vi "Execute (Multiple result with rows).vi"(8 "error in (no error)":errorcluster, 10 "SQL":string, 11 "PQ Connection in":refnum<class "PQ Connection.lvclass">) -> (0 "error out":errorcluster, 1 "Results with Rows returned":refnum<class "PQ Result.lvclass">[](array[class]), 3 "PQ Connection out":refnum<class "PQ Connection.lvclass">)   [LabVIEW 2015, in "PQ Connection.lvclass"]
uses:
  PQ Connection.lvclass
  Result/PQ Result.lvclass
  PQ Connection.lvclass/PQ Connection.ctl
  Result/PQ Result.lvclass/PQ Result.ctl
  libpq.dll
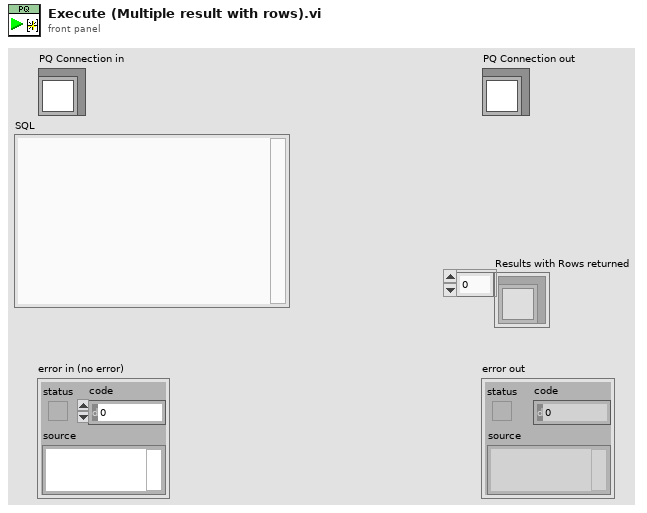
[diagram p1: front panel]
types:
  T1 = typedef "PQ Result.lvclass/Result Status.ctl" = enum32{"PGRES_EMPTY_QUERY", "PGRES_COMMAND_OK", "PGRES_TUPLES_OK", "PGRES_COPY_OUT", "PGRES_COPY_IN", "PGRES_BAD_RESPONSE", "PGRES_NONFATAL_ERROR", "PGRES_FATAL_ERROR", "PGRES_COPY_BOTH", "PGRES_SINGLE_TUPLE"}
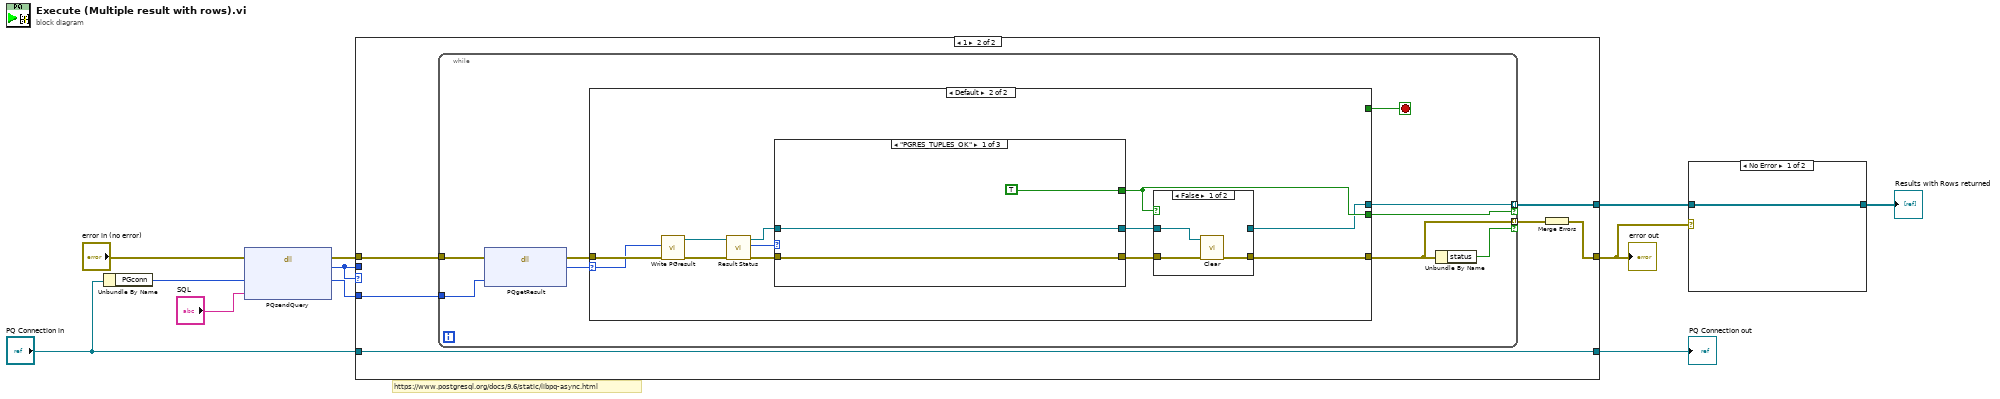
[diagram p0: block diagram]
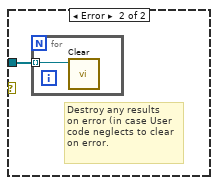
[diagram p2: hidden frame]
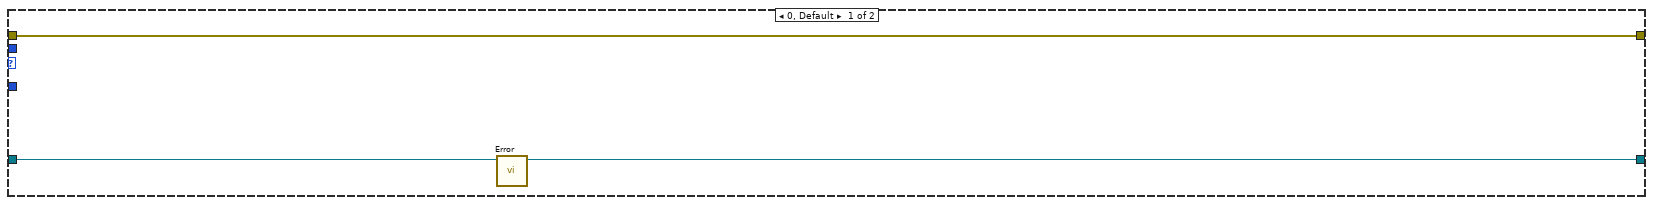
[diagram p3: hidden frame]
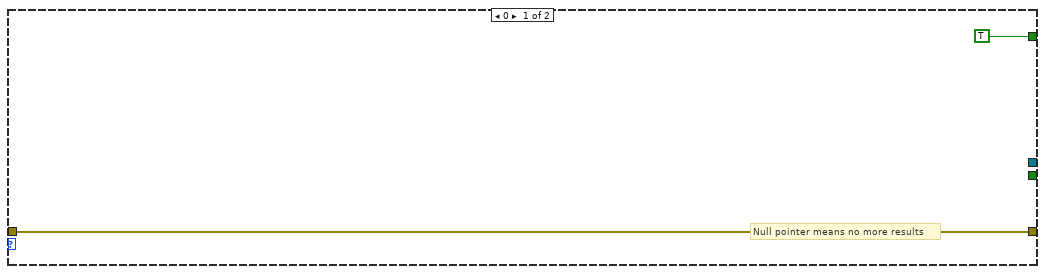
[diagram p4: hidden frame]
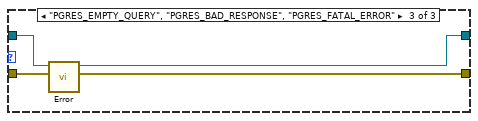
[diagram p6: hidden frame]
diagram:
  # "https://www.postgresql.org/docs/9.6/static/libpq-async.html"
  n1 = Unbundle By Name("PQ Connection in") -> ("PGconn"=w10:u32)
  n2 = dll-call lib="C:/PQ/Connection/libpq.dll" fn="PQsendQuery" ("libpq.*:PQexec")(error in="error in (no error)", "PGconn"=w10, "command"="SQL") -> (error out=w9:errorcluster, "OK?"=w7:u32, "PGconn"=w4:u32)  [unwired: 3 in, 1 out]
  n3 = case shown="1" w7 {
    tunnel: w9 -> [w12 w20]
    tunnel: w7 -> [_ _]
    tunnel: [_ w19] -> w2
    tunnel: [w12 w15] -> w1
    tunnel: "PQ Connection in" -> [w14 w16]
    tunnel: [w13 w16] -> w5
    tunnel: w4 -> [_ w17]
    frame 0, Default {
      n4 = call "Error.vi"("PQ Connection in"=w14) -> ("PQ Connection out"=w13:refnum<class "PQ Connection.lvclass">)  [unwired: 9 in, 1 out]
    }
    frame 1 {
      n5 = while {
        tunnel: [w27] -> w19 mode=indexing if=w28
        tunnel: w17 -> [w29]
        tunnel: w20 -> [w24]
        tunnel: [w22] -> w18 mode=indexing if=w21
        stop <- w25 stop-if-true
        n6 = dll-call lib="C:/PQ/Connection/libpq.dll" fn="PQgetResult" ("libpq.*:PQexec")(error in=w24, "PGconn"=w29) -> (error out=w23:errorcluster, "PQresult"=w26:u32)  [unwired: 3 in, 1 out]
        n7 = case shown="Default" w26 {
          selector: w26 -> [_ w32]
          tunnel: w23 -> [w31 w43]
          tunnel: [_ w42] -> w28
          tunnel: [_ w40] -> w27
          tunnel: [w31 w38] -> w22
          tunnel: [TRUE _] -> w25
          frame 0 {
            # "Null pointer means no more results"
          }
          frame Default {
            n8 = call "Write PGresult.vi"("error in (no error)"=w43, "PGresult"=w32) -> ("error out"=w36:errorcluster, "PQ Result  out"=w37:refnum<class "PQ Result.lvclass">)  [unwired: 8 in]
            n9 = call "Result Status.vi"("error in (no error)"=w36, "PQ Result in"=w37) -> ("error out"=w33:errorcluster, "Result Status"=w35:T1, "PQ Result out"=w34:refnum<class "PQ Result.lvclass">)  [unwired: 7 in]
            n10 = case shown="\"PGRES_TUPLES_OK\"" w35 {
              tunnel: [w45 w47 w49] -> w41
              tunnel: w34 -> [w45 w47 w52]
              tunnel: w33 -> [w46 w48 w51]
              tunnel: [w46 w48 w50] -> w39
              tunnel: [TRUE _ _] -> w42
              frame "PGRES_TUPLES_OK" {
              }
              frame Default {
                # "No results, but not error"
              }
              frame "PGRES_EMPTY_QUERY", "PGRES_BAD_RESPONSE", "PGRES_FATAL_ERROR" {
                n11 = call "Error.vi"("error in (no error)"=w51, "PQ Result  In"=w52) -> ("error out"=w50:errorcluster, "PQ Result"=w49:refnum<class "PQ Result.lvclass">)  [unwired: 8 in]
              }
            }
            n12 = case shown="False" w42 {
              tunnel: w41 -> [w55 w57]
              tunnel: [_ w57] -> w40
              tunnel: w39 -> [w54 w56]
              tunnel: [w53 w56] -> w38
              frame False {
                n13 = call "Clear.vi"("error in (no error)"=w54, "PQ Result  in"=w55) -> ("error out"=w53:errorcluster)  [unwired: 9 in]
              }
              frame True {
              }
            }
          }
        }
        n14 = Unbundle By Name(w22) -> ("status"=w21:bool)
      }
      n15 = Merge Errors(w18) -> (w15:errorcluster)
    }
  }
  "error out" <- w1
  "PQ Connection out" <- w5
  n16 = case shown="No Error" w1 {
    tunnel: [w58 _] -> w3
    tunnel: w2 -> [w58 w59]
    frame No Error {
    }
    frame Error {
      # "Destroy any results\non error (in case User\ncode neglects to clear\non error."
      n17 = for {
        tunnel: w59 -> [w60] mode=indexing
        n18 = call "Clear.vi"("PQ Result  in"=w60) -> ()  [unwired: 10 in, 1 out]
      }
    }
  }
  "Results with Rows returned" <- w3
